vi "IV curve.vi"() -> ()   [LabVIEW 2017]
uses:
  <instrlib>/Keithley 24XX/Public/Data/Read (Single Point).vi
  <vilib>/Utility/file.llb/Write Delimited Spreadsheet (DBL).vi
  <instrlib>/Keithley 24XX/Keithley 24XX.lvlib
panel:
  in  "Number of loops":i32=10
  in  "Delay Time (s)":dbl=0.5
  out "Next Voltage":dbl
  out "Voltage":sgl
  out "XY Graph 2":cluster{sgl[], dbl[]}(graph)
  out "Time vs. Resistance":cluster{sgl[], dbl[]}(graph)
  in  "Save to:":path
  in  "Reset":bool
  in  "Voltage (V) Manual":dbl
  out "error out":errorcluster
  in  "error in (no error)":errorcluster
  in  "stop":bool
  in  "Start Measurment":bool
  in  "Voltage steps size (V)":dbl
  in  "Max Positive Voltage (V)":dbl
  in  "Keithley (GPIB:20)":refnum<visa-resource-name>
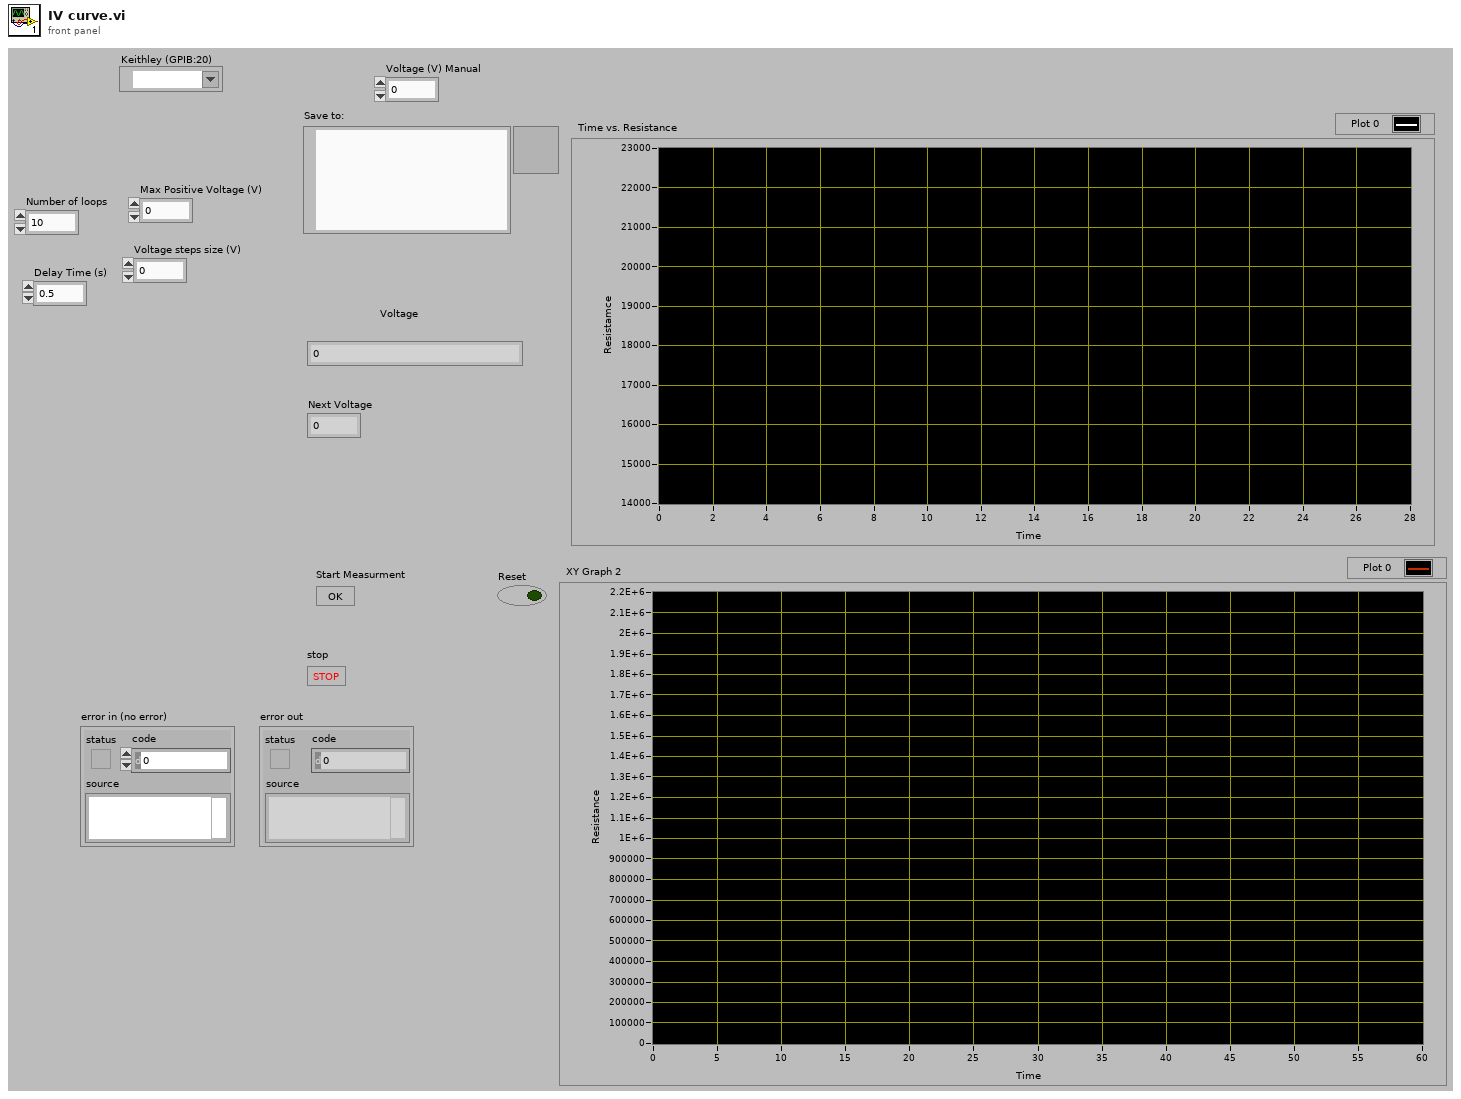
[diagram p1: front panel]
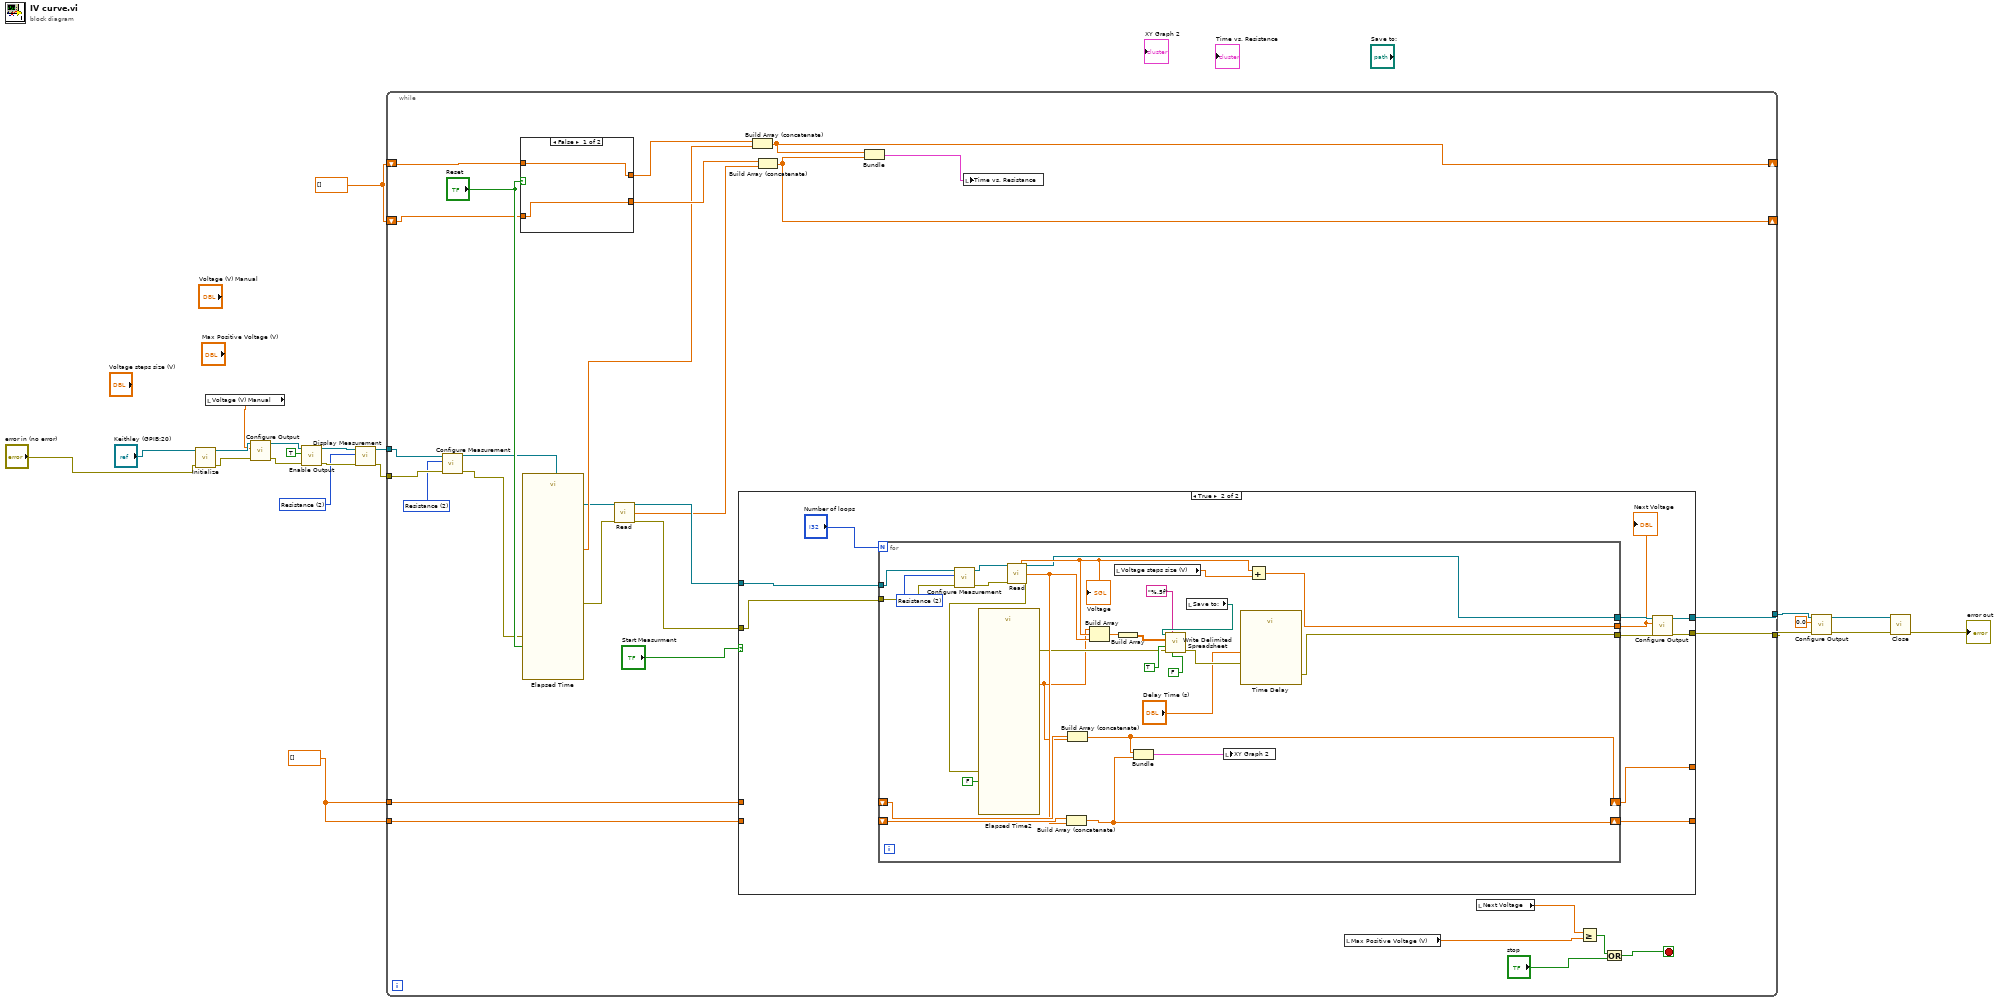
[diagram p0: block diagram]
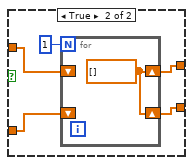
[diagram p2: hidden frame]
diagram:
  w1 = sgl[] []
  w3 = sgl[] []
  w13 = u16 2 items=["Voltage", "Current", "Resistance"] ("Displayed Measurement (0: Voltage)")
  n1 = call <instrlib>:"Initialize.vi"("error in (no error)"="error in (no error)", "VISA resource name"="Keithley (GPIB:20)") -> ("error out"=w19:errorcluster, "VISA resource name out"=w14:refnum<visa-resource-name>)  [unwired: 8 in]
  n2 = local read "Voltage (V) Manual"() -> (w2:dbl)
  n3 = call <instrlib>:"Configure Output.vi"("error in (no error)"=w19, "Output Level (0)"=w2, "VISA resource name"=w14) -> ("error out"=w18:errorcluster, "VISA resource name out"=w15:refnum<visa-resource-name>)  [unwired: 7 in]
  n4 = call <instrlib>:"Enable Output.vi"("error in (no error)"=w18, "Enable Output (T: Enable)"=TRUE, "VISA resource name"=w15) -> ("error out"=w17:errorcluster, "VISA resource name out"=w16:refnum<visa-resource-name>)  [unwired: 7 in]
  n5 = call <instrlib>:"Display Measurement.vi"("error in (no error)"=w17, "Displayed Measurement (0: Voltage)"=w13, "VISA resource name"=w16) -> ("error out"=w10:errorcluster, "VISA resource name out"=w11:refnum<visa-resource-name>)  [unwired: 7 in]
  n6 = while {
    tunnel: w11 -> [w48]
    tunnel: w10 -> [w47]
    tunnel: [w42] -> w9
    tunnel: [w41] -> w8
    shift-right: [w36] -> _
    shift-left: w3 -> [w39]
    shift-right: [w35] -> _
    shift-left: w3 -> [w38]
    tunnel: w1 -> [w23]
    tunnel: w1 -> [w22]
    stop <- w28 stop-if-true
    w37 = u16 2 items=["Volts", "Current", "Resistance"] ("Function (0: Volts)")
    n7 = call <instrlib>:"Configure Measurement.vi"("error in (no error)"=w47, "Function (0: Volts)"=w37, "VISA resource name"=w48) -> ("error out"=w24:errorcluster, "VISA resource name out"=w25:refnum<visa-resource-name>)  [unwired: 7 in]
    n8 = case shown="False" "Reset" {
      tunnel: w39 -> [w51 w55]
      tunnel: w38 -> [w50 w54]
      tunnel: [w51 w52] -> w45
      tunnel: [w50 w53] -> w44
      frame False {
      }
      frame True {
        n9 = for {
          N: 1 -> [_]
          shift-right: [w57] -> w53
          shift-left: w54 -> [_]
          shift-right: [w57] -> w52
          shift-left: w55 -> [_]
          w57 = sgl[] []
        }
      }
    }
    n10 = call "Elapsed Time"("Reset"="Reset", "error in (no error)"=w24) -> ("Elapsed Time (s)"=w34:dbl, "error out"=w46:errorcluster)  [unwired: 10 in, 6 out]
    n11 = call-poly <instrlib>:"Read.vi"("VISA resource name"=w25, "error in (no error)"=w46) -> ("VISA resource name out"=w43:refnum<visa-resource-name>, "Resistance"=w33:sgl, "error out"=w31:errorcluster)  [unwired: 7 in, 4 out]
    n12 = case shown="True" "Start Measurment" {
      tunnel: w43 -> [w60 w64]
      tunnel: w31 -> [w61 w65]
      tunnel: [w61 w68] -> w42
      tunnel: [w60 w69] -> w41
      tunnel: [w59 w63] -> _
      tunnel: [w58 w62] -> _
      tunnel: w23 -> [w59 _]
      tunnel: w22 -> [w58 _]
      frame False {
      }
      frame True {
        n13 = for {
          N: "Number of loops" -> [_]
          tunnel: w64 -> [w99]
          tunnel: w65 -> [w98]
          shift-right: [w91] -> w63
          shift-left: _ -> [w94]
          shift-right: [w92] -> w62
          shift-left: _ -> [w93]
          tunnel: [w75] -> w71
          tunnel: [w76] -> w70
          tunnel: [w74] -> w66
          w97 = u16 2 items=["Volts", "Current", "Resistance"] ("Function (0: Volts)")
          n14 = call <instrlib>:"Configure Measurement.vi"("error in (no error)"=w98, "Function (0: Volts)"=w97, "VISA resource name"=w99) -> ("error out"=w95:errorcluster, "VISA resource name out"=w96:refnum<visa-resource-name>)  [unwired: 7 in]
          n15 = call-poly <instrlib>:"Read.vi"("VISA resource name"=w96, "error in (no error)"=w95) -> ("Voltage"=w89:sgl, "VISA resource name out"=w76:refnum<visa-resource-name>, "Resistance"=w80:sgl, "error out"=w79:errorcluster)  [unwired: 7 in, 3 out]
          "Voltage" <- w89
          n16 = call "Elapsed Time2"("Reset"=FALSE, "error in (no error)"=w79) -> ("Elapsed Time (s)"=w77:dbl, "error out"=w78:errorcluster)  [unwired: 10 in, 6 out]
          n17 = Build Array (concatenate)(w93, w80) -> (w92:sgl[])
          n18 = Build Array (concatenate)(w94, w77) -> (w91:dbl[])
          n19 = Build Array(w77, w89, w80) -> (w88:dbl[])
          n20 = local read "Voltage steps size (V)"() -> (w90:dbl)
          n21 = Build Array(w88) -> (w86:dbl[][])
          n22 = Bundle(w91, w92) -> (w87:cluster{dbl[], sgl[]})  [unwired: 1 in]
          n23 = local read "Save to:"() -> (w84:path)
          n24 = call-poly <vilib>:"Write Delimited Spreadsheet.vi"("file path (dialog if empty)"=w84, "format (%.3f)"="%.5f", "2D data"=w86, "append to file? (new file:F)"=TRUE, "error in (no error)"=w78, "transpose? (no:F)"=FALSE) -> ("error out"=w85:errorcluster)  [unwired: 8 in, 1 out]
          n25 = local write "XY Graph 2"(w87) -> ()
          n26 = call "Time Delay"("error in (no error)"=w85, "Delay Time (s)"="Delay Time (s)") -> ("error out"=w75:errorcluster)  [unwired: 9 in]
          n27 = Add(x=w89, y=w90) -> (x+y=w74:dbl)
        }
        "Next Voltage" <- w66
        n28 = call <instrlib>:"Configure Output.vi"("error in (no error)"=w71, "Output Level (0)"=w66, "VISA resource name"=w70) -> ("error out"=w68:errorcluster, "VISA resource name out"=w69:refnum<visa-resource-name>)  [unwired: 7 in]
      }
    }
    n29 = Build Array (concatenate)(w45, w34) -> (w36:dbl[])
    n30 = Build Array (concatenate)(w44, w33) -> (w35:sgl[])
    n31 = Bundle(w36, w35) -> (w32:cluster{dbl[], sgl[]})  [unwired: 1 in]
    n32 = local write "Time vs. Resistance"(w32) -> ()
    n33 = local read "Max Positive Voltage (V)"() -> (w29:dbl)
    n34 = local read "Next Voltage"() -> (w27:dbl)
    n35 = Greater Or Equal?(x=w27, y=w29) -> (x >= y?=w30:bool)
    n36 = Or(x=w30, y="stop") -> (x .or. y?=w28:bool)
  }
  n37 = call <instrlib>:"Configure Output.vi"("error in (no error)"=w9, "Output Level (0)"=0.0, "VISA resource name"=w8) -> ("error out"=w7:errorcluster, "VISA resource name out"=w5:refnum<visa-resource-name>)  [unwired: 7 in]
  n38 = call <instrlib>:"Close.vi"("error in (no error)"=w7, "VISA resource name"=w5) -> ("error out"=→"error out":errorcluster)  [unwired: 9 in]
